vi "Update Intensity Chart History.vi"(8 "error in (no error)":errorcluster, 10 "Y":dbl[](array[numeric]), 11 "Array in":dbl[][](array[numeric])) -> (0 "error out":errorcluster, 3 "Array out":dbl[][](array[numeric]))   [LabVIEW 2017]
doc: "Updates the intensity chart history."
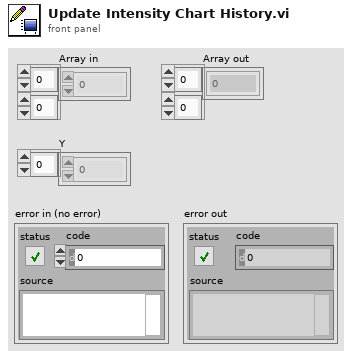
[diagram p1: front panel]
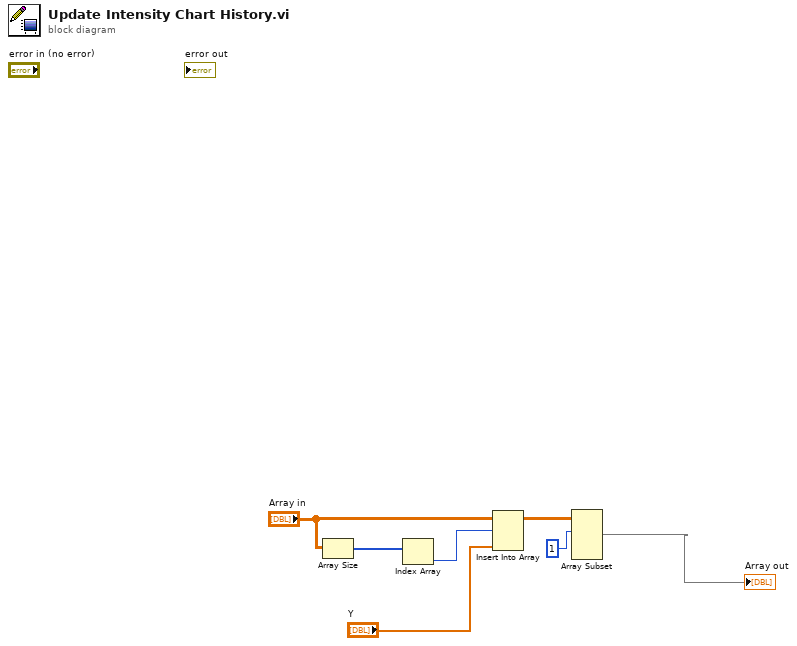
[diagram p0: block diagram]
diagram:
  n1 = Array Size(array="Array in") -> (size(s)=w1:i32[])
  n2 = Index Array(array=w1) -> (element=w2:i32)  [unwired: 1 in]
  n3 = Insert Into Array(array="Array in", index (row)=w2, new element="Y") -> (w3:dbl[][])  [unwired: 1 in]
  n4 = Array Subset(array=w3, index (row)=1 ("index")) -> (→"Array out":dbl[][])  [unwired: 3 in]
